vi "SetPrecision.vi"(8 "error in":errorcluster, 10 "Precision":u8=6, 11 "RealMeasure in":refnum<class "RealMeasure.lvclass">) -> (0 "error out":errorcluster, 3 "RealMeasure out":refnum<class "RealMeasure.lvclass">)   [LabVIEW 2021, in "ProligentXMLGenerator.lvlib" / "RealMeasure.lvclass"]
doc: "Defines the actual date where the step run ended.\n\nThis value is restricted to \"1900-01-01T00:00:00Z\" -\"2100-01-01T00:00:00Z\"."
uses:
  RealMeasure.lvclass
  RealMeasure.lvclass/RealMeasure.ctl
  MeasureLimit/MeasureLimit.lvclass
  RealMeasureLimit/RealMeasureLimit.lvclass
  Base/String_4000/String_4000.lvclass
  Base/UnsignedByte/UnsignedByte.lvclass
  Base/Decimal/Decimal.lvclass
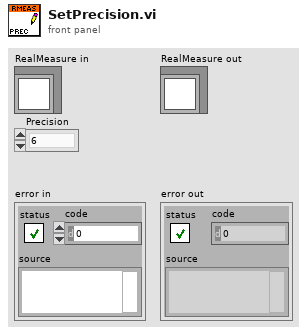
[diagram p1: front panel]
types:
  T1 = typedef "ProligentXMLGenerator.lvlib/RealMeasure.lvclass/Data.ctl" = cluster{"Value":refnum<class "Decimal.lvclass">, "Precision":refnum<class "UnsignedByte.lvclass">}
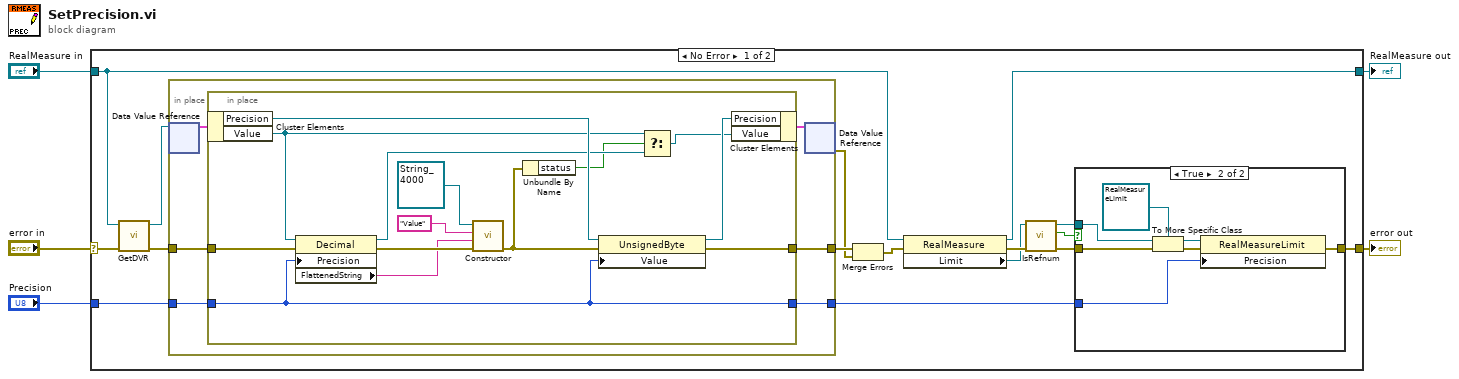
[diagram p0: block diagram]
diagram:
  n1 = case shown="No Error" "error in" {
    selector: "error in" -> [w20 w50]
    tunnel: "RealMeasure in" -> [w7 w51]
    tunnel: [w8 w50] -> w3
    tunnel: "Precision" -> [w16 _]
    tunnel: [w15 w51] -> w1
    frame No Error {
      n2 = call "GetDVR.vi"("error in"=w20, "RealMeasure"=w7) -> ("error out"=w19:errorcluster, "DVRReference"=w21:refnum<data-value>)  [unwired: 8 in]
      n3 = in-place "In Place Element Structure" {
        in-place-border: w19 -> [w33]
        in-place-border: [w35] -> w18
        in-place-border: w16 -> [w34]
        in-place-border: [w30] -> w14
        n4 = in-place-dvr #1(w21) -> (w32:T1)  [unwired: 1 out]
        n5 = in-place "In Place Element Structure" {
          in-place-border: [w49] -> w35
          in-place-border: w34 -> [w41]
          in-place-border: w33 -> [w42]
          in-place-border: [w41] -> w30
          n6 = in-place-cluster #2(w32) -> ("Precision"=w48:refnum<class "UnsignedByte.lvclass">, "Value"=w39:refnum<class "Decimal.lvclass">)
          n7 = property on="Property Node" class="Decimal"(reference=w39, error in=w42, "Precision"=w41) -> (reference out=w40:refnum<class "Decimal.lvclass">, error out=w45:errorcluster, "FlattenedString"=w43:string)
          n8 = call-dynamic "Constructor.vi"("error in"=w45, "Value"=w43, "Name"="Value", "String in"=refnum<class "String_4000.lvclass"> refnum ("ProligentResultProcessor:String_4000")) -> ("error out"=w36:errorcluster)  [unwired: 6 in, 1 out]
          n9 = Unbundle By Name(w36) -> ("status"=w38:bool)
          n10 = property on="Property Node" class="UnsignedByte"(reference=w48, error in=w36, "Value"=w41) -> (reference out=w47:refnum<class "UnsignedByte.lvclass">, error out=w49:errorcluster)
          n11 = Select(t=w39, s=w38, f=w40) -> (s? t:f=w37:refnum<class "Decimal.lvclass">)
          n12 = in-place-cluster #2("Precision"=w47, "Value"=w37) -> (w31:T1)
        }
        n13 = in-place-dvr #1(w31) -> (w6:errorcluster)  [unwired: 1 out]
      }
      n14 = Merge Errors(w18, w6) -> (w17:errorcluster)
      n15 = property on="Property Node" class="RealMeasure"(reference=w7, error in=w17) -> (reference out=w15:refnum<class "RealMeasure.lvclass">, error out=w13:errorcluster, "Limit"=w10:refnum<class "MeasureLimit.lvclass">)
      n16 = call "IsRefnum.vi"("error in"=w13, "MeasureLimit in"=w10) -> ("error out"=w12:errorcluster, "IsRefnum"=w11:bool, "MeasureLimit out"=w9:refnum<class "MeasureLimit.lvclass">)  [unwired: 7 in]
      n17 = case shown="True" w11 {
        tunnel: w14 -> [_ w24]
        tunnel: w12 -> [w22 w29]
        tunnel: w9 -> [_ w28]
        tunnel: [w22 w27] -> w8
        frame False {
        }
        frame True {
          n18 = To More Specific Class(target class=refnum<class "RealMeasureLimit.lvclass"> refnum ("ProligentResultProcessor:RealMeasureLimit"), reference=w28, error in=w29) -> (specific class reference=w26:refnum<class "RealMeasureLimit.lvclass">, error out=w25:errorcluster)
          n19 = property on="Property Node" class="RealMeasureLimit"(reference=w26, error in=w25, "Precision"=w24) -> (error out=w27:errorcluster)  [unwired: 1 out]
        }
      }
    }
    frame Error {
    }
  }
  "error out" <- w3
  "RealMeasure out" <- w1
